vi "Probe.vi"(11 "Engine out":refnum<class "Engine.lvclass">) -> (2 "Value String":string, 3 "Boolean":bool)   [LabVIEW 2020, in "GLF.lvlib" / "Engine.lvclass"]
uses:
  Engine.lvclass
  Engine.lvclass/Engine.ctl
  Metrics--cluster.ctl
  <vilib>/Saukko/LV SDL3/Sources/SDL3/Events/EventType--enum.ctl
  <vilib>/Saukko/LV SDL3/Sources/SDL3/Events/Events.lvlib
panel:
  out "Unhandled Events":cluster{"EventType":T1, "Count":u64}[](array[cluster])
  out "Metrics":T2
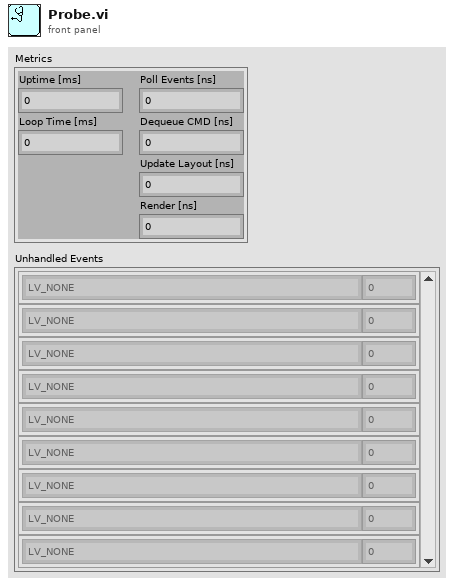
[diagram p1: front panel]
types:
  T1 = typedef "SDL3.lvlib/Events.lvlib/EventType--enum.ctl" = enum16{"LV_NONE", "LV_UNSUPPORTED", "SDL_EVENT_QUIT", "SDL_EVENT_LOCALE_CHANGED", "SDL_EVENT_SYSTEM_THEME_CHANGED", "SDL_EVENT_DISPLAY_ORIENTATION", "SDL_EVENT_DISPLAY_ADDED", "SDL_EVENT_DISPLAY_REMOVED", "SDL_EVENT_DISPLAY_MOVED", "SDL_EVENT_DISPLAY_DESKTOP_MODE_CHANGED", "SDL_EVENT_DISPLAY_CURRENT_MODE_CHANGED", "SDL_EVENT_DISPLAY_CONTENT_SCALE_CHANGED", "SDL_EVENT_WINDOW_SHOWN", "SDL_EVENT_WINDOW_HIDDEN", "SDL_EVENT_WINDOW_EXPOSED", "SDL_EVENT_WINDOW_MOVED", "SDL_EVENT_WINDOW_RESIZED", "SDL_EVENT_WINDOW_PIXEL_SIZE_CHANGED", "SDL_EVENT_WINDOW_METAL_VIEW_RESIZED", "SDL_EVENT_WINDOW_MINIMIZED", "SDL_EVENT_WINDOW_MAXIMIZED", "SDL_EVENT_WINDOW_RESTORED", "SDL_EVENT_WINDOW_MOUSE_ENTER", "SDL_EVENT_WINDOW_MOUSE_LEAVE", "SDL_EVENT_WINDOW_FOCUS_GAINED", "SDL_EVENT_WINDOW_FOCUS_LOST", "SDL_EVENT_WINDOW_CLOSE_REQUESTED", "SDL_EVENT_WINDOW_HIT_TEST", "SDL_EVENT_WINDOW_ICCPROF_CHANGED", "SDL_EVENT_WINDOW_DISPLAY_CHANGED", "SDL_EVENT_WINDOW_DISPLAY_SCALE_CHANGED", "SDL_EVENT_WINDOW_SAFE_AREA_CHANGED", "SDL_EVENT_WINDOW_OCCLUDED", "SDL_EVENT_WINDOW_ENTER_FULLSCREEN", "SDL_EVENT_WINDOW_LEAVE_FULLSCREEN", "SDL_EVENT_WINDOW_DESTROYED", "SDL_EVENT_WINDOW_HDR_STATE_CHANGED", "SDL_EVENT_KEY_DOWN", "SDL_EVENT_KEY_UP", "SDL_EVENT_TEXT_EDITING", "SDL_EVENT_TEXT_INPUT", "SDL_EVENT_KEYMAP_CHANGED", "SDL_EVENT_KEYBOARD_ADDED", "SDL_EVENT_KEYBOARD_REMOVED", "SDL_EVENT_TEXT_EDITING_CANDIDATES", "SDL_EVENT_MOUSE_MOTION", "SDL_EVENT_MOUSE_BUTTON_DOWN", "SDL_EVENT_MOUSE_BUTTON_UP", "SDL_EVENT_MOUSE_WHEEL", "SDL_EVENT_MOUSE_ADDED", "SDL_EVENT_MOUSE_REMOVED", "SDL_EVENT_JOYSTICK_AXIS_MOTION", "SDL_EVENT_JOYSTICK_BALL_MOTION", "SDL_EVENT_JOYSTICK_HAT_MOTION", "SDL_EVENT_JOYSTICK_BUTTON_DOWN", "SDL_EVENT_JOYSTICK_BUTTON_UP", "SDL_EVENT_JOYSTICK_ADDED", "SDL_EVENT_JOYSTICK_REMOVED", "SDL_EVENT_JOYSTICK_BATTERY_UPDATED", "SDL_EVENT_JOYSTICK_UPDATE_COMPLETE", "SDL_EVENT_GAMEPAD_AXIS_MOTION", "SDL_EVENT_GAMEPAD_BUTTON_DOWN", "SDL_EVENT_GAMEPAD_BUTTON_UP", "SDL_EVENT_GAMEPAD_ADDED", "SDL_EVENT_GAMEPAD_REMOVED", "SDL_EVENT_GAMEPAD_REMAPPED", "SDL_EVENT_GAMEPAD_TOUCHPAD_DOWN", "SDL_EVENT_GAMEPAD_TOUCHPAD_MOTION", "SDL_EVENT_GAMEPAD_TOUCHPAD_UP", "SDL_EVENT_GAMEPAD_SENSOR_UPDATE", "SDL_EVENT_GAMEPAD_UPDATE_COMPLETE", "SDL_EVENT_GAMEPAD_STEAM_HANDLE_UPDATED", "SDL_EVENT_FINGER_DOWN", "SDL_EVENT_FINGER_UP", "SDL_EVENT_FINGER_MOTION", "SDL_EVENT_CLIPBOARD_UPDATE", "SDL_EVENT_DROP_FILE", "SDL_EVENT_DROP_TEXT", "SDL_EVENT_DROP_BEGIN", "SDL_EVENT_DROP_COMPLETE", "SDL_EVENT_DROP_POSITION", "SDL_EVENT_AUDIO_DEVICE_ADDED", "SDL_EVENT_AUDIO_DEVICE_REMOVED", "SDL_EVENT_AUDIO_DEVICE_FORMAT_CHANGED", "SDL_EVENT_SENSOR_UPDATE", "SDL_EVENT_PEN_PROXIMITY_IN", "SDL_EVENT_PEN_PROXIMITY_OUT", "SDL_EVENT_PEN_DOWN", "SDL_EVENT_PEN_UP", "SDL_EVENT_PEN_BUTTON_DOWN", "SDL_EVENT_PEN_BUTTON_UP", "SDL_EVENT_PEN_MOTION", "SDL_EVENT_PEN_AXIS", "SDL_EVENT_CAMERA_DEVICE_ADDED", "SDL_EVENT_CAMERA_DEVICE_REMOVED", "SDL_EVENT_CAMERA_DEVICE_APPROVED", "SDL_EVENT_CAMERA_DEVICE_DENIED", "SDL_EVENT_RENDER_TARGETS_RESET", "SDL_EVENT_RENDER_DEVICE_RESET", "SDL_EVENT_POLL_SENTINEL", "SDL_EVENT_USER"}
  T2 = typedef "GLF.lvlib/Engine.lvclass/Metrics--cluster.ctl" = cluster{"Uptime [ms]":u64, "Loop Time [ms]":u64, "Poll Events [ns]":u64, "Dequeue CMD [ns]":u64, "Update Layout [ns]":u64, "Render [ns]":u64}
  T3 = typedef "GLF.lvlib/Engine.lvclass/DVR--cluster.ctl" = cluster{"CMD Queue":T4, "Config":T5, "Ctxt":T7, "Metrics":T2, "Window Instances":map{T8, refnum<class "Window.lvclass">}, "Debug":T9}
  T4 = typedef "GLF.lvlib/Engine.lvclass/Command--queue.ctl" = refnum<queue>
  T5 = typedef "GLF.lvlib/Engine.lvclass/Config--cluster.ctl" = cluster{"Quit On Last Window Closed":bool, "VSync":T6, "FPS Target":dbl}
  T6 = typedef "GLF.lvlib/Engine.lvclass/VSync--enum.ctl" = enum16{"Disabled", "Enabled", "Adaptative"}
  T7 = typedef "GLF.lvlib/Engine.lvclass/Context--cluster.ctl" = cluster{"Ticks Begin":u64, "VSync Enabled":bool}
  T8 = typedef "SDL3.lvlib/Video.lvlib/WindowID--integer.ctl" = u32
  T9 = typedef "GLF.lvlib/Engine.lvclass/Debug--cluster.ctl" = cluster{"Unhandled Events":map{T1, u64}}
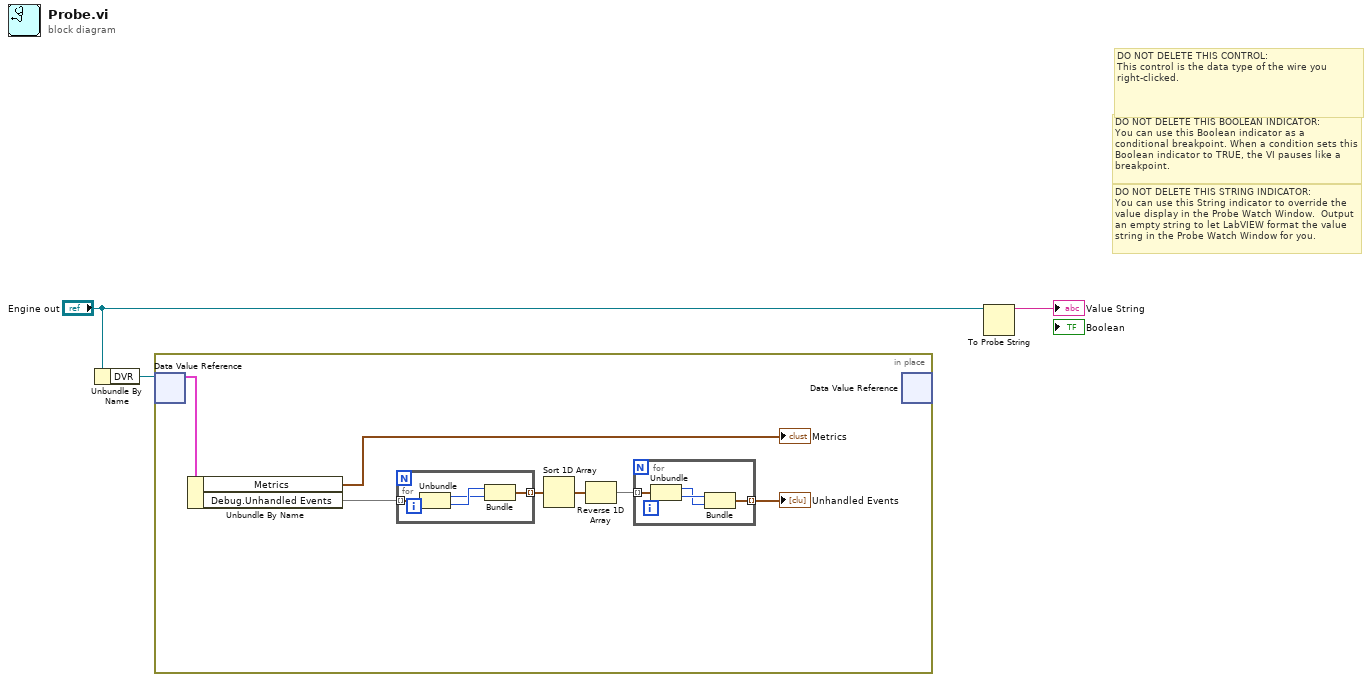
[diagram p0: block diagram]
diagram:
  # "DO NOT DELETE THIS STRING INDICATOR: \nYou can use this String indicator to override the value display in the Probe Watch Window.  Output an empty string to let LabVIEW format the value string in the Probe Watch Window for you."
  # "DO NOT DELETE THIS BOOLEAN INDICATOR: \nYou can use this Boolean indicator as a conditional breakpoint. When a condition sets this Boolean indicator to TRUE, the VI pauses like a breakpoint."
  # "DO NOT DELETE THIS CONTROL: \nThis control is the data type of the wire you right-clicked."
  n1 = Unbundle By Name("Engine out") -> ("DVR"=w1:refnum<data-value>)
  n2 = in-place {
    n3 = in-place-dvr #1(w1) -> (w10:T3)  [unwired: 1 out]
    n4 = Unbundle By Name(w10) -> ("Metrics"=→"Metrics":T2, "Debug.Unhandled Events"=w9:map{T1, u64})
    n5 = for {
      tunnel: w9 -> [w18] mode=indexing
      tunnel: [w15] -> w8 mode=indexing
      n6 = Unbundle(w18) -> ("EventType"=w16:T1, "Count"=w17:u64)
      n7 = Bundle("Count"=w17, "EventType"=w16) -> (w15:cluster{"Count":u64, "EventType":T1})  [unwired: 1 in]
    }
    n8 = Sort 1D Array(array=w8) -> (sorted array=w7:cluster{"Count":u64, "EventType":T1}[])
    n9 = Reverse 1D Array(array=w7) -> (reversed array=w6:cluster{"Count":u64, "EventType":T1}[])
    n10 = for {
      tunnel: w6 -> [w14] mode=indexing
      tunnel: [w11] -> w4 mode=indexing
      n11 = Unbundle(w14) -> ("Count"=w12:u64, "EventType"=w13:T1)
      n12 = Bundle("EventType"=w13, "Count"=w12) -> (w11:cluster{"EventType":T1, "Count":u64})  [unwired: 1 in]
    }
    "Unhandled Events" <- w4
    n13 = in-place-dvr #1() -> ()  [unwired: 1 in, 2 out]
  }
  n14 = To Probe String(7:"Engine out") -> (3:→"Value String":string)  [unwired: 2 in, 1 out]
